vi "Oscilator waveform generator.vi"(4 "Number of Samples":i32=1000, 6 "signal type":T1(ring), 7 "phase in":dbl format="%.2p", 8 "error in":errorcluster, 9 "Frequency":dbl=10.0 format="%0.2p", 10 "Amplitude":dbl=1.0 format="%0.2p", 11 "DAQdx task in":refnum<k21>) -> (0 "error out":errorcluster, 1 "MAQdx sampling rate":dbl, 2 "Oscilator waveform":waveform(dbl), 3 "DAQdx task out":refnum<k21>, 5 "phase out":dbl format="%.2p")   [LabVIEW 2014]
uses:
  <vilib>/measure/NI_MABase.lvlib
  <resource>/objmgr/daqmx.rc
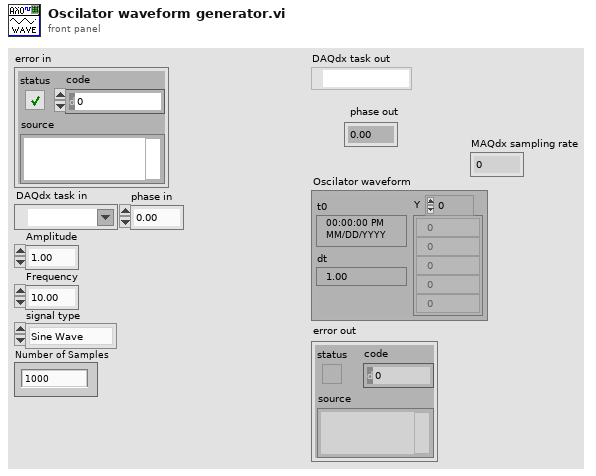
[diagram p1: front panel]
types:
  T1 = enum16{"Sine Wave", "Triangle Wave", "Square Wave", "Sawtooth Wave"}
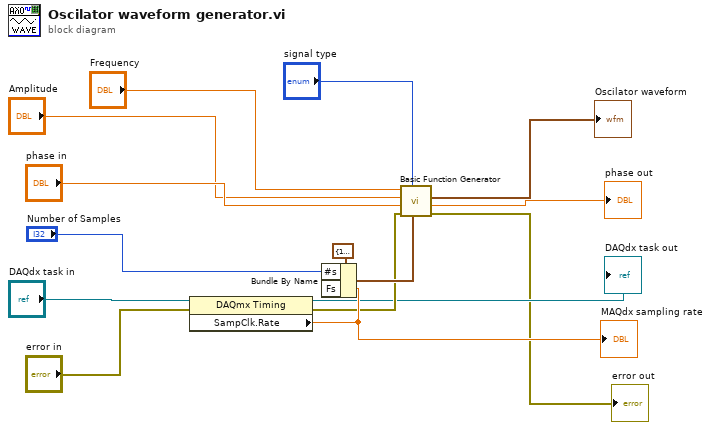
[diagram p0: block diagram]
diagram:
  n1 = property class="DAQmx Timing"(reference="DAQdx task in", error in="error in") -> (reference out=→"DAQdx task out":refnum<k21>, error out=w12:errorcluster, "SampClk.Rate"=w14:dbl)
  "MAQdx sampling rate" <- w14
  n2 = Bundle By Name(cluster=cluster{"Fs":dbl, "#s":dbl} {"Fs"=1000.0, "#s"=1000.0} ("sampling info"), "#s"="Number of Samples", "Fs"=w14) -> (w13:cluster{"Fs":dbl, "#s":dbl})
  n3 = call <vilib>:"Basic Function Generator.vi"("sampling info"=w13, "signal type"="signal type", "error in (no error)"=w12, "phase"="phase in", "amplitude"="Amplitude", "frequency"="Frequency") -> ("error out"=→"error out":errorcluster, "phase out"=→"phase out":dbl, "signal out"=→"Oscilator waveform":waveform(dbl))  [unwired: 3 in]
